vi "Get VI Reference.vi"(8 "error in (no error)":errorcluster, 11 "JKI SM in":refnum<class "JKI SM.lvclass">) -> (0 "error out":errorcluster, 2 "VI":refnum<vi>, 3 "JKI SM out":refnum<class "JKI SM.lvclass">)   [LabVIEW 2020, in "JKI State Machine API.lvlib" / "JKI SM.lvclass"]
uses:
  JKI SM.lvclass
  JKI SM.lvclass/JKI SM.ctl
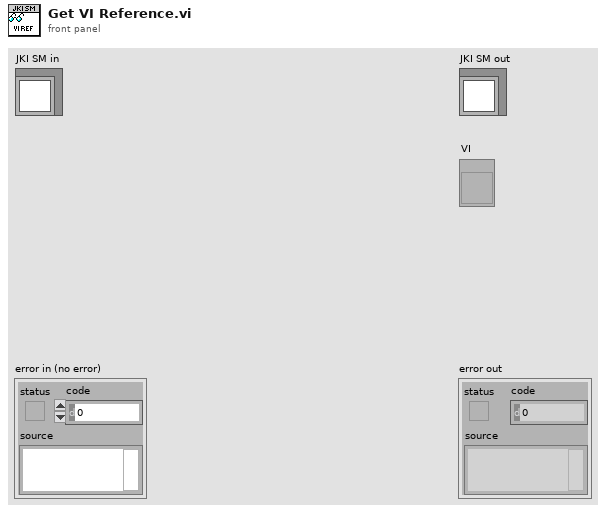
[diagram p1: front panel]
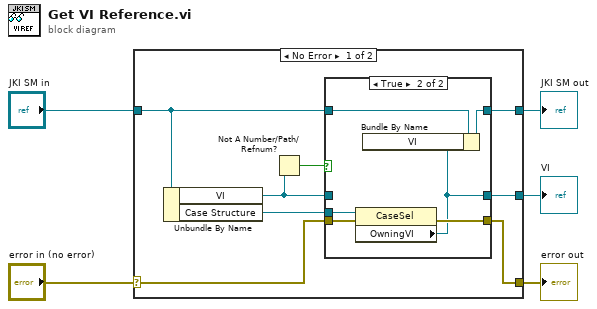
[diagram p0: block diagram]
diagram:
  n1 = case shown="No Error" "error in (no error)" {
    selector: "error in (no error)" -> [w9 w23]
    tunnel: [w8 w23] -> w4
    tunnel: [w11 w24] -> w2
    tunnel: "JKI SM in" -> [w12 w24]
    tunnel: [w7 _] -> w1
    frame No Error {
      n2 = Unbundle By Name(w12) -> ("VI"=w6:refnum<vi>, "Case Structure"=w10:refnum<vi>)
      n3 = Not A Number/Path/Refnum?(number/path/refnum=w6) -> (NaN/Path/Refnum?=w13:bool)
      n4 = case shown="True" w13 {
        tunnel: w12 -> [w16 w22]
        tunnel: [w16 w21] -> w11
        tunnel: w10 -> [_ w20]
        tunnel: w9 -> [w15 w19]
        tunnel: [w15 w18] -> w8
        tunnel: [w14 w17] -> w7
        tunnel: w6 -> [w14 _]
        frame False {
        }
        frame True {
          n5 = property class="CaseSel"(reference=w20, error in=w19) -> (error out=w18:errorcluster, "OwningVI"=w17:refnum<vi>)  [unwired: 1 out]
          n6 = Bundle By Name(cluster=w22, "VI"=w17) -> (w21:refnum<class "JKI SM.lvclass">)
        }
      }
    }
    frame Error {
    }
  }
  "error out" <- w4
  "JKI SM out" <- w2
  "VI" <- w1
